vi "Event Delete SW.vi"(8 "error in (no error)":errorcluster, 11 "[MV] Key Generator in":refnum<class "[MV] Key Generator.lvclass">) -> (0 "error out":errorcluster, 3 "[MV] Key Generator out":refnum<class "[MV] Key Generator.lvclass">)   [LabVIEW 2020, in "[MV] Key Generator.lvlib" / "[MV] Key Generator.lvclass"]
uses:
  [MV] Key Generator.lvclass
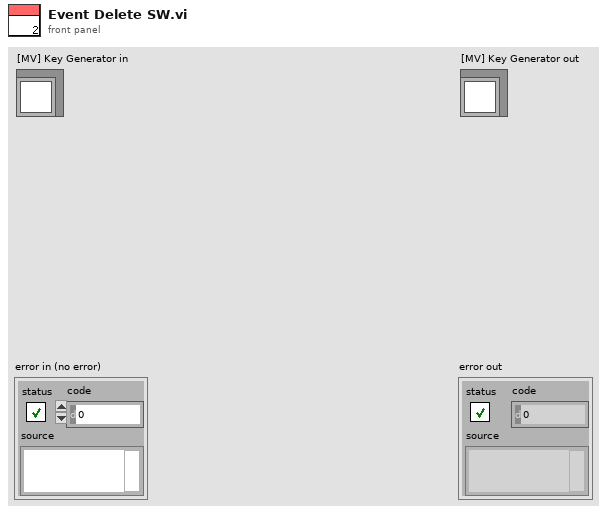
[diagram p1: front panel]
types:
  T1 = map{string, cluster{"private":string, "public":string}}
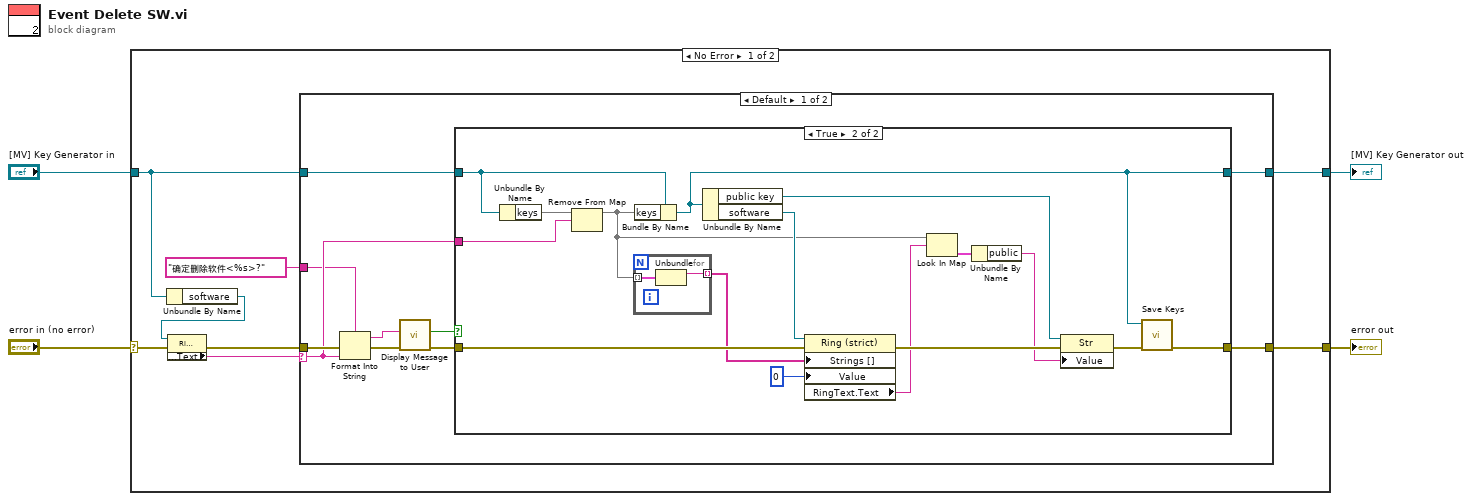
[diagram p0: block diagram]
diagram:
  n1 = case shown="No Error" "error in (no error)" {
    selector: "error in (no error)" -> [w12 w46]
    tunnel: [w8 w46] -> w3
    tunnel: [w5 w45] -> w1
    tunnel: "[MV] Key Generator in" -> [w6 w45]
    frame No Error {
      n2 = Unbundle By Name(w6) -> ("software"=w11:refnum<vi>)
      n3 = property class="Ring (strict)"(reference=w11, error in=w12) -> (error out=w9:errorcluster, "RingText.Text"=w10:string)  [unwired: 1 out]
      n4 = case shown="Default" w10 {
        selector: w10 -> [w16 _]
        tunnel: w9 -> [w22 w44]
        tunnel: [w14 w44] -> w8
        tunnel: "确定删除软件<%s>?" ("format string") -> [w15 _]
        tunnel: w6 -> [w17 w43]
        tunnel: [w13 w43] -> w5
        frame Default {
          n5 = Format Into String(format string=w15, error in=w22, w16) -> (resulting string=w20:string, error out=w21:errorcluster)  [unwired: 1 in]
          n6 = call "Display Message to User"("error in (no error)"=w21, "Message"=w20) -> ("error out"=w18:errorcluster, "确定"=w19:bool)  [unwired: 8 in]
          n7 = case shown="True" w19 {
            tunnel: w18 -> [w24 w36]
            tunnel: w17 -> [w23 w38]
            tunnel: w16 -> [_ w27]
            tunnel: [w24 w39] -> w14
            tunnel: [w23 w37] -> w13
            frame False {
            }
            frame True {
              n8 = Unbundle By Name(w38) -> ("keys"=w40:T1)
              n9 = Remove From Map(10:w27, 11:w40) -> (3:w34:T1)  [unwired: 2 out]
              n10 = for {
                tunnel: w34 -> [w42] mode=indexing
                tunnel: [w41] -> w28 mode=indexing
                n11 = Unbundle(w42) -> ("name"=w41:string)  [unwired: 1 out]
              }
              n12 = Bundle By Name(cluster=w38, "keys"=w34) -> (w37:refnum<class "[MV] Key Generator.lvclass">)
              n13 = Unbundle By Name(w37) -> ("public key"=w32:refnum<vi>, "software"=w35:refnum<vi>)
              n14 = property class="Ring (strict)"(reference=w35, error in=w36, "Strings []"=w28, "Value"=u16 0) -> (error out=w33:errorcluster, "RingText.Text"=w25:string)  [unwired: 1 out]
              n15 = Look In Map(map=w34, key=w25) -> (value=w30:cluster{"private":string, "public":string})  [unwired: 1 in, 1 out]
              n16 = Unbundle By Name(w30) -> ("public"=w29:string)
              n17 = property class="Str"(reference=w32, error in=w33, "Value"=w29) -> (error out=w31:errorcluster)  [unwired: 1 out]
              n18 = call "Save Keys.vi"("error in (no error)"=w31, "[MV] Key Generator in"=w37) -> ("error out"=w39:errorcluster)  [unwired: 8 in, 1 out]
            }
          }
        }
        frame "" {
        }
      }
    }
    frame Error {
    }
  }
  "error out" <- w3
  "[MV] Key Generator out" <- w1
